vi "Dialog Test.vi"() -> ()   [LabVIEW 2009]
uses:
  Controls/methodCall.ctl
  Controls/methodResponse.ctl
  XML-RPC Parser/GetScalarValue/ValueAsString.vi
panel:
  in  "methodResponse":T1
  out "error out":errorcluster
  in  "methodCall":T2
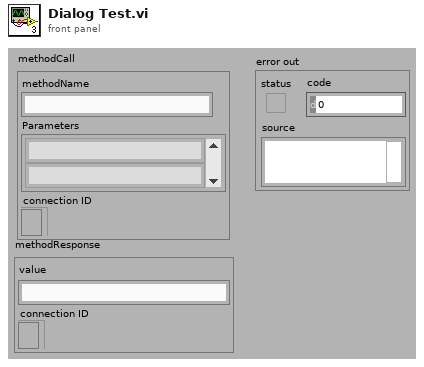
[diagram p1: front panel]
types:
  T1 = typedef "methodResponse.ctl" = cluster{"value":string, "connection ID":refnum<k5>}
  T2 = typedef "methodCall.ctl" = cluster{"methodName":string, "Parameters":string[], "connection ID":refnum<k5>}
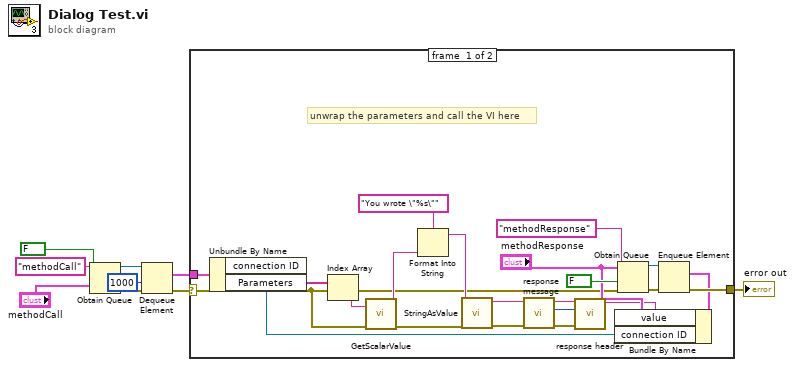
[diagram p0: block diagram]
diagram:
  n1 = Obtain Queue(name (unnamed)="methodCall", element data type="methodCall", create if not found? (T)=FALSE) -> (queue out=w9:refnum<queue>, error out=w8:errorcluster)  [unwired: 2 in, 1 out]
  n2 = Dequeue Element(queue=w9, timeout in ms (-1)=1000, error in (no error)=w8) -> (element=w3:T2, error out=w4:errorcluster)  [unwired: 2 out]
  n3 = case shown="No Error" w4 {
    selector: w4 -> [w10 w32]
    tunnel: w3 -> [w31 _]
    tunnel: [w27 w32] -> w2
    frame #0 {
      # "unwrap the parameters and call the VI here"
      n4 = Unbundle By Name(w31) -> ("connection ID"=w11:refnum<k5>, "Parameters"=w26:string[])
      n5 = Index Array(array=w26) -> (element=w25:string)  [unwired: 1 in]
      n6 = call-poly "GetScalarValue.vi"("error in (no error)"=w10, "Parameter"=w25) -> ("error out"=w24:errorcluster, "value"=w18:string)  [unwired: 8 in]
      n7 = Format Into String(format string="You wrote \"%s\"", w18) -> (resulting string=w17:string)  [unwired: 2 in, 1 out]
      n8 = call "StringAsValue.vi"("error in"=w24, "scalar value (string)"=w17) -> ("error out"=w22:errorcluster, "scalar string"=w23:string)  [unwired: 8 in]
      n9 = call "response message.vi"("error in"=w22, "params (formatted)"=w23) -> ("error out"=w19:errorcluster, "length"=w20:i32, "response"=w21:string)  [unwired: 7 in]
      n10 = call "response header.vi"("error in"=w19, "Content-Length"=w20, "Content String"=w21) -> ("response string"=w13:string)  [unwired: 7 in, 1 out]
      n11 = Bundle By Name(cluster="methodResponse", "value"=w13, "connection ID"=w11) -> (w12:T1)
      n12 = Obtain Queue(name (unnamed)="methodResponse", element data type="methodResponse", create if not found? (T)=FALSE, error in (no error)=w10) -> (queue out=w28:refnum<queue>, error out=w29:errorcluster)  [unwired: 1 in, 1 out]
      n13 = Enqueue Element(queue=w28, element=w12, error in (no error)=w29) -> (error out=w27:errorcluster)  [unwired: 1 in, 2 out]
    }
    frame #1 {
    }
  }
  "error out" <- w2
